vi "Configure Trigger (Edge Burst).vi"(6 "Edge Slope (0: Positive)":i32(ring) items=["Positive", "Negative"], 7 "Idle Time (5E-7 S)":dbl=5e-07, 8 "error in (no error)":errorcluster, 9 "Edge Count (1)":i32=1, 10 "Source Channel (0: Channel 1)":i32(ring) items=["Channel 1"=0, "Channel 2"=1, "Channel 3"=2, "Channel 4"=3, "D0"=13, "D1"=14, "D2"=15, "D3"=16, "D4"=17, "D5"=18, "D6"=19, "D7"=20, "D8"=21, "D9"=22, "D10"=23, "D11"=24, "D12"=25, "D13"=26, "D14"=27, "D15"=28], 11 "VISA resource name":refnum<visa-resource-name>) -> (0 "error out":errorcluster, 3 "VISA resource name out":refnum<visa-resource-name>)   [LabVIEW 2023, in "Keysight-DSQx3014T.lvlib"]
doc: "Configures the edge burst trigger mode."
uses:
  Keysight-DSQx3014T.lvlib
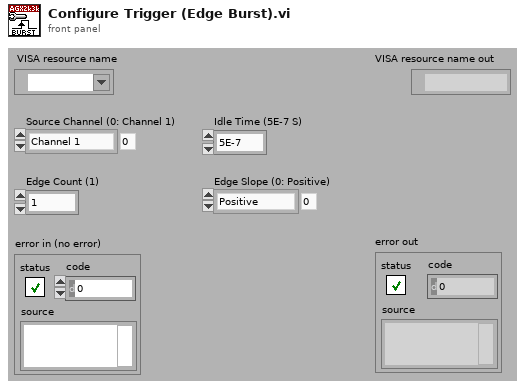
[diagram p1: front panel]
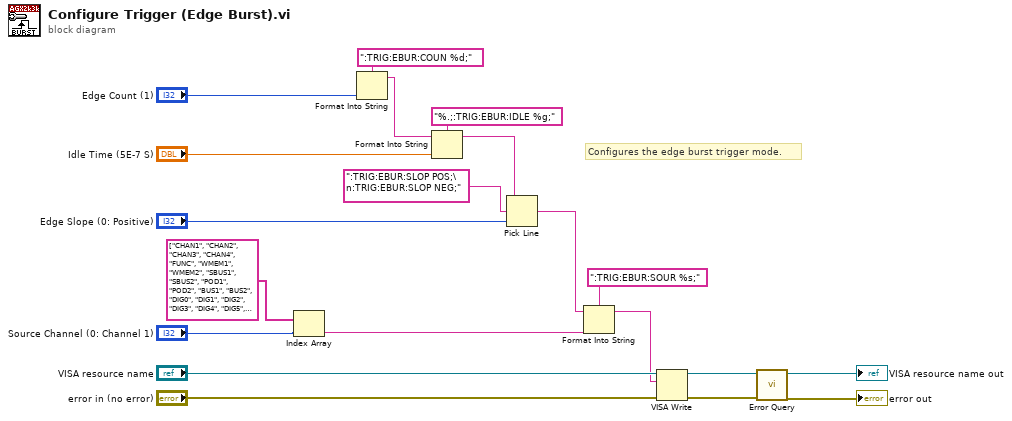
[diagram p0: block diagram]
diagram:
  # "Configures the edge burst trigger mode."
  n1 = Index Array(array=string[] ["CHAN1", "CHAN2", "CHAN3", "CHAN4", "FUNC", "WMEM1", "WMEM2", "SBUS1", "SBUS2", "POD1", "POD2", "BUS1", "BUS2", "DIG0", "DIG1", "DIG2", "DIG3", "DIG4", "DIG5", "DIG6", "DIG7", "DIG8", "DIG9", "DIG10", "DIG11", "DIG12", "DIG13", "DIG14", "DIG15", "EXT", "LINE", "WGEN"], index="Source Channel (0: Channel 1)") -> (element=w1:string)
  n2 = Format Into String(format string=":TRIG:EBUR:COUN %d;", "Edge Count (1)") -> (resulting string=w18:string)  [unwired: 2 in, 1 out]
  n3 = Format Into String(format string="%.;:TRIG:EBUR:IDLE %g;", initial string=w18, "Idle Time (5E-7 S)") -> (resulting string=w13:string)  [unwired: 1 in, 1 out]
  n4 = Pick Line(string ("")=w13, multi-line string=":TRIG:EBUR:SLOP POS;\n:TRIG:EBUR:SLOP NEG;", line index="Edge Slope (0: Positive)") -> (output string=w5:string)
  n5 = Format Into String(format string=":TRIG:EBUR:SOUR %s;", initial string=w5, w1) -> (resulting string=w6:string)  [unwired: 1 in, 1 out]
  n6 = VISA Write(VISA resource name="VISA resource name", write buffer=w6, error in (no error)="error in (no error)") -> (VISA resource name out=w10:refnum<visa-resource-name>, error out=w9:errorcluster)  [unwired: 1 out]
  n7 = call "Error Query.vi"("error in (no error)"=w9, "VISA resource name"=w10) -> ("error out"=→"error out":errorcluster, "VISA resource name out"=→"VISA resource name out":refnum<visa-resource-name>)  [unwired: 8 out]
